vi "Vendor Request Data.vi"(8 "error in (no error)":errorcluster, 11 "CallVendorRequest in":refnum<class "CallVendorRequest.lvclass">) -> (0 "error out":errorcluster, 2 "Vendor Request Data JSON":string, 3 "CallVendorRequest out":refnum<class "CallVendorRequest.lvclass">)   [LabVIEW 2020, in "obs-websocket.lvlib" / "CallVendorRequest.lvclass"]
uses:
  CallVendorRequest.lvclass
  CallVendorRequest.lvclass/CallVendorRequest.ctl
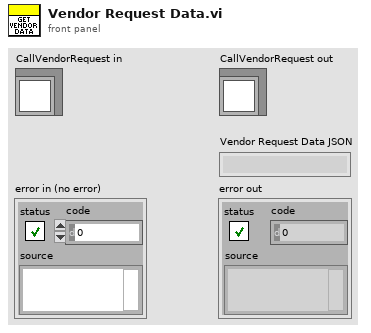
[diagram p1: front panel]
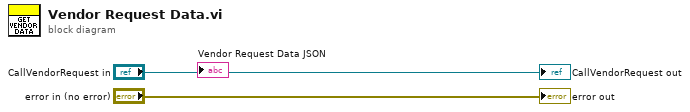
[diagram p0: block diagram]
diagram:
  "error out" <- "error in (no error)"
  "CallVendorRequest out" <- "CallVendorRequest in"
